vi "DT_Triangle Manager_Get Adj Ghost.vi"(8 "cur point idx":i32, 9 "cur base point idx":i32, 10 "cur triangle":i32, 11 "Triangles In":i32[][](array[numeric])) -> (0 "next point idx":i32, 1 "next base point idx":i32, 2 "next triangle":i32)   [LabVIEW 2017, in "NI_AAL_Geometry.lvlib"]
uses:
  <vilib>/Analysis/NI_AAL_Geometry.lvlib
  <vilib>/Analysis/geometry.llb/DT_Triangle Manager_Get Ghost Point.vi
  <vilib>/Analysis/geometry.llb/DT_Triangle Manager_Get Oppo Point.vi
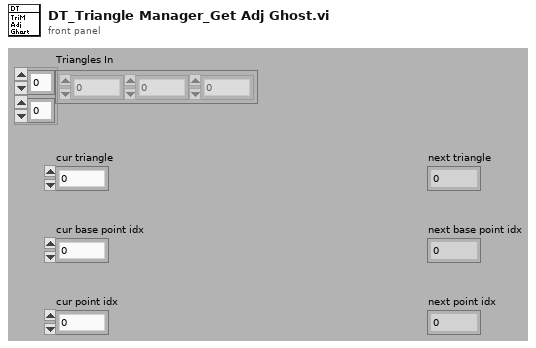
[diagram p1: front panel]
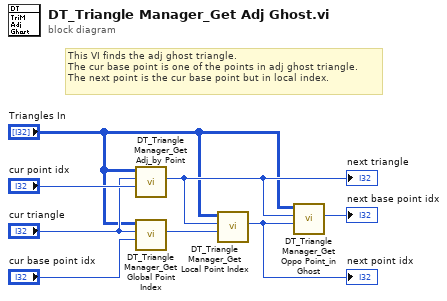
[diagram p0: block diagram]
diagram:
  # "This VI finds the adj ghost triangle.\nThe cur base point is one of the points in adj ghost triangle.\nThe next point is the cur base point but in local index."
  n1 = call <vilib>:"DT_Triangle Manager_Get Adj_by Point.vi"("point idx"="cur point idx", "triangle"="cur triangle", "Triangles In"="Triangles In") -> ("adj triangle"=w4:i32)  [unwired: 8 out]
  "next triangle" <- w4
  n2 = call <vilib>:"DT_Triangle Manager_Get Global Point Index.vi"("local idx"="cur base point idx", "triangle"="cur triangle", "Triangles"="Triangles In") -> ("global idx"=w8:i32)  [unwired: 8 out]
  n3 = call <vilib>:"DT_Triangle Manager_Get Local Point Index.vi"("global idx"=w8, "triangle"=w4, "Triangles"="Triangles In") -> ("local idx"=w3:i32)  [unwired: 8 out]
  "next point idx" <- w3
  n4 = call <vilib>:"DT_Triangle Manager_Get Oppo Point_in Ghost.vi"("point idx"=w3, "triangle"=w4, "Triangles"="Triangles In") -> ("opposite point idx"=→"next base point idx":i32)  [unwired: 8 out]
